vi "PIO.Write U32 Array.vi"(8 "error in (no error)":errorcluster, 9 "values":u32[](array[numeric]), 10 "offset":u32 format="%.0x", 11 "GE 5565PIORC in":refnum<class "GE 5565PIORC Old.lvclass">) -> (0 "error out":errorcluster, 3 "GE 5565PIORC out":refnum<class "GE 5565PIORC Old.lvclass">)   [LabVIEW 2016, in "GE 5565PIORC Old.lvclass"]
uses:
  GE 5565PIORC Old.lvclass
  GE 5565PIORC Old.lvclass/GE 5565PIORC Old.ctl
  <vilib>/Instr/_visa.llb/VISA Register Access Address Space.ctl
  Change Endianness (U32).vi
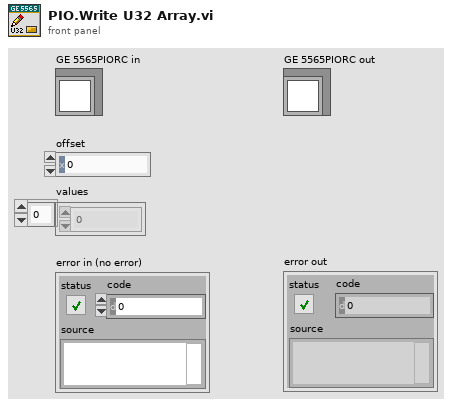
[diagram p1: front panel]
types:
  T1 = typedef "VISA Register Access Address Space.ctl" = u16
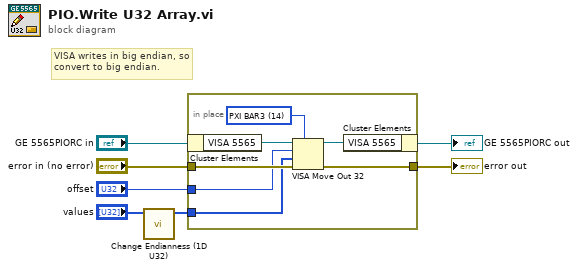
[diagram p0: block diagram]
diagram:
  # "VISA writes in big endian, so convert to big endian."
  n1 = call "Change Endianness (1D U32).vi"("array in"="values") -> ("byte-reversed array out"=w1:u32[])  [unwired: 10 in]
  n2 = in-place {
    in-place-border: "error in (no error)" -> [w14]
    in-place-border: [w13] -> w6
    in-place-border: "offset" -> [w10]
    in-place-border: w1 -> [w8]
    w11 = T1 14 items=["VXI/VME A16"=1, "VXI/VME A24"=2, "VXI/VME A32"=3, "VXI/VME A64"=4, "PXI Memory Allocations"=9, "PXI Configuration"=10, "PXI BAR0"=11, "PXI BAR1"=12, "PXI BAR2"=13, "PXI BAR3"=14, "PXI BAR4"=15, "PXI BAR5"=16] ("Address Space")
    n3 = in-place-cluster #1("GE 5565PIORC in") -> ("VISA 5565"=w12:refnum<visa-resource-name>)
    n4 = VISA Move Out 32(7:w11, 8:w14, 9:w8, 10:w10, 11:w12) -> (0:w13:errorcluster, 3:w9:refnum<visa-resource-name>)
    n5 = in-place-cluster #1("VISA 5565"=w9) -> (→"GE 5565PIORC out":refnum<class "GE 5565PIORC Old.lvclass">)
  }
  "error out" <- w6
